vi "SpreadsheetFGV.vi"(6 "Message Ref":refnum<vi>, 7 "FGV Control":T1=enum."Init", 8 "Error In":errorcluster, 10 "Check -in Time":timestamp, 11 "Student ID":i32) -> (0 "Error Out":errorcluster, 1 "Checked In?":bool, 2 "Names":string[](array[string]), 3 "Message":string, 4 "Elapsed Time":i32)   [LabVIEW 2017]
uses:
  Controls/CSVFGVStates.ctl
  <vilib>/Utility/file.llb/Write To Spreadsheet File (string).vi
  <vilib>/Utility/file.llb/Read From Spreadsheet File (string).vi
panel:
  out "Output 2D Data":string[][](array[string])
  in  "CheckedInOutColumn":i32=3
  out "Checked In":string
  out "all rows":string[][](array[string])
  in  "Replacement":string
  in  "Student Names":i32(listbox)
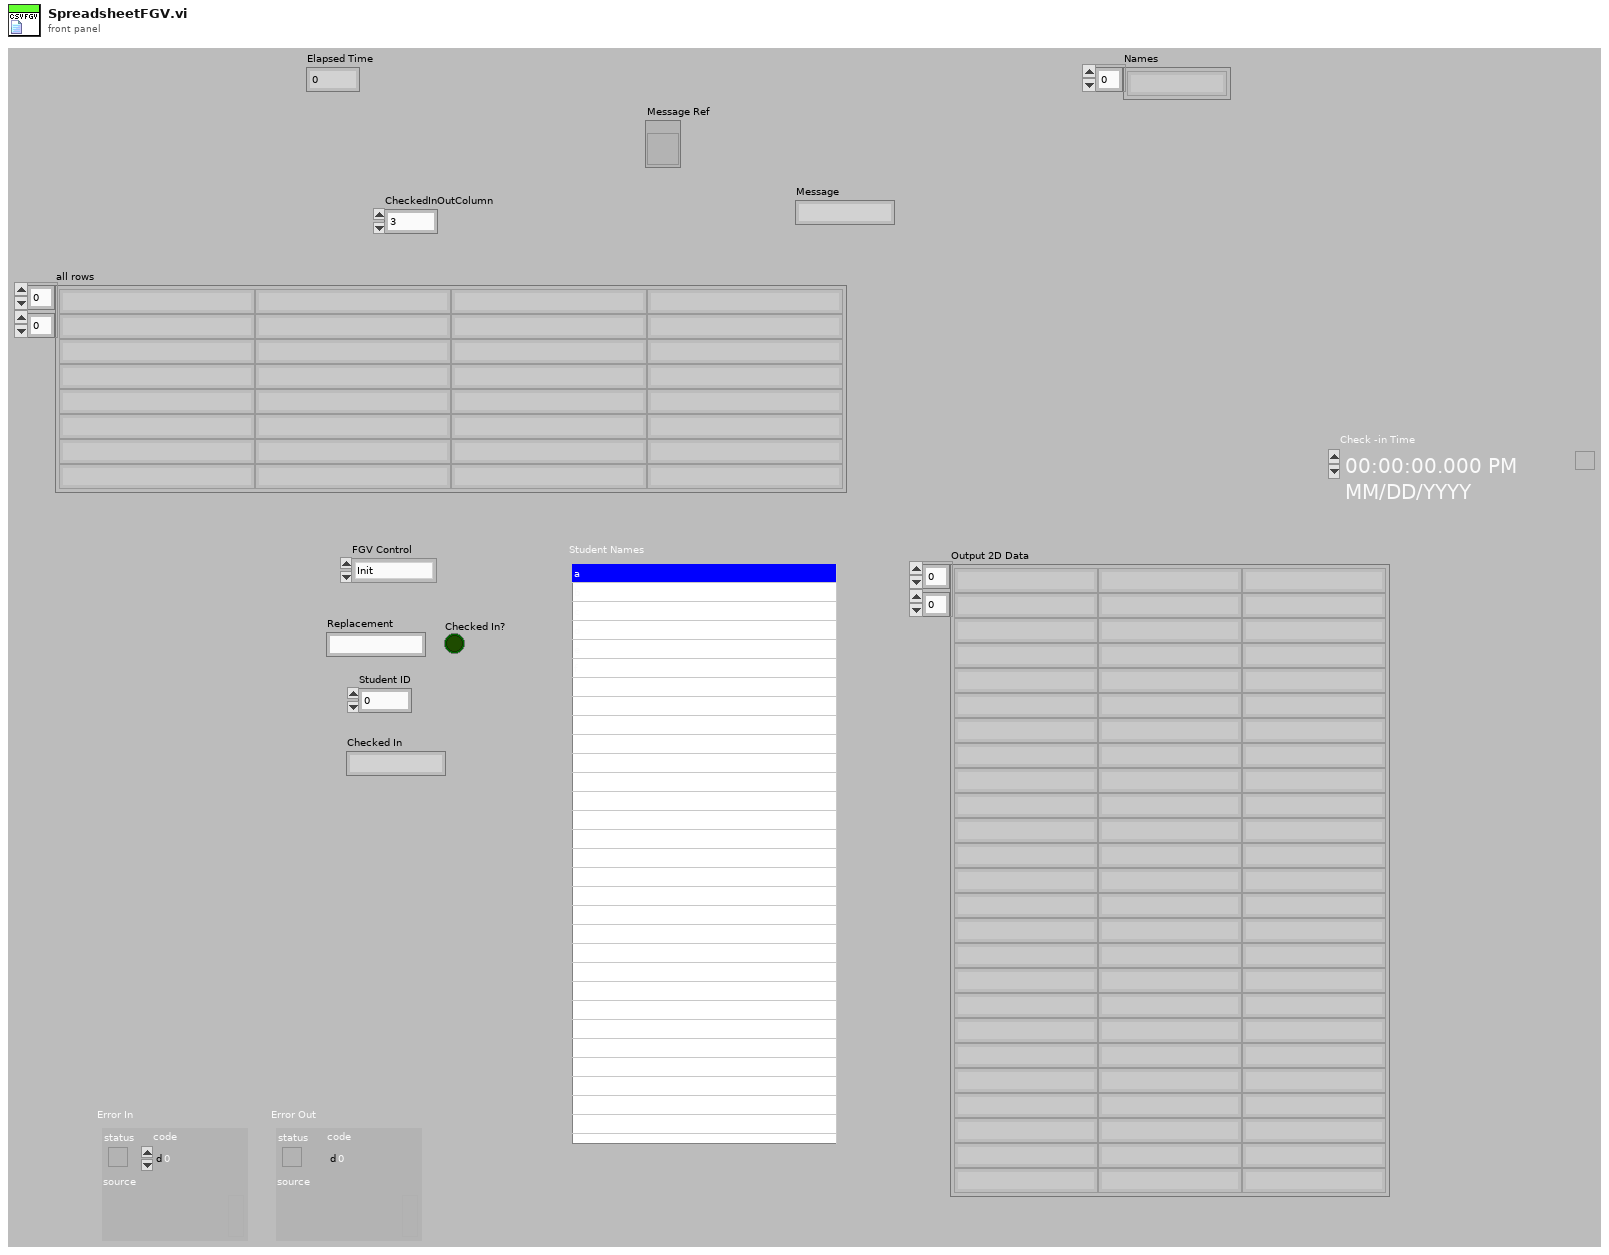
[diagram p1: front panel]
types:
  T1 = typedef "CSVFGVStates.ctl" = enum16{"Quit", "Init", "Sort", "Disable Camera", "Check In", "Check Out", "Check Status", "Read CSV", "Close Out"}
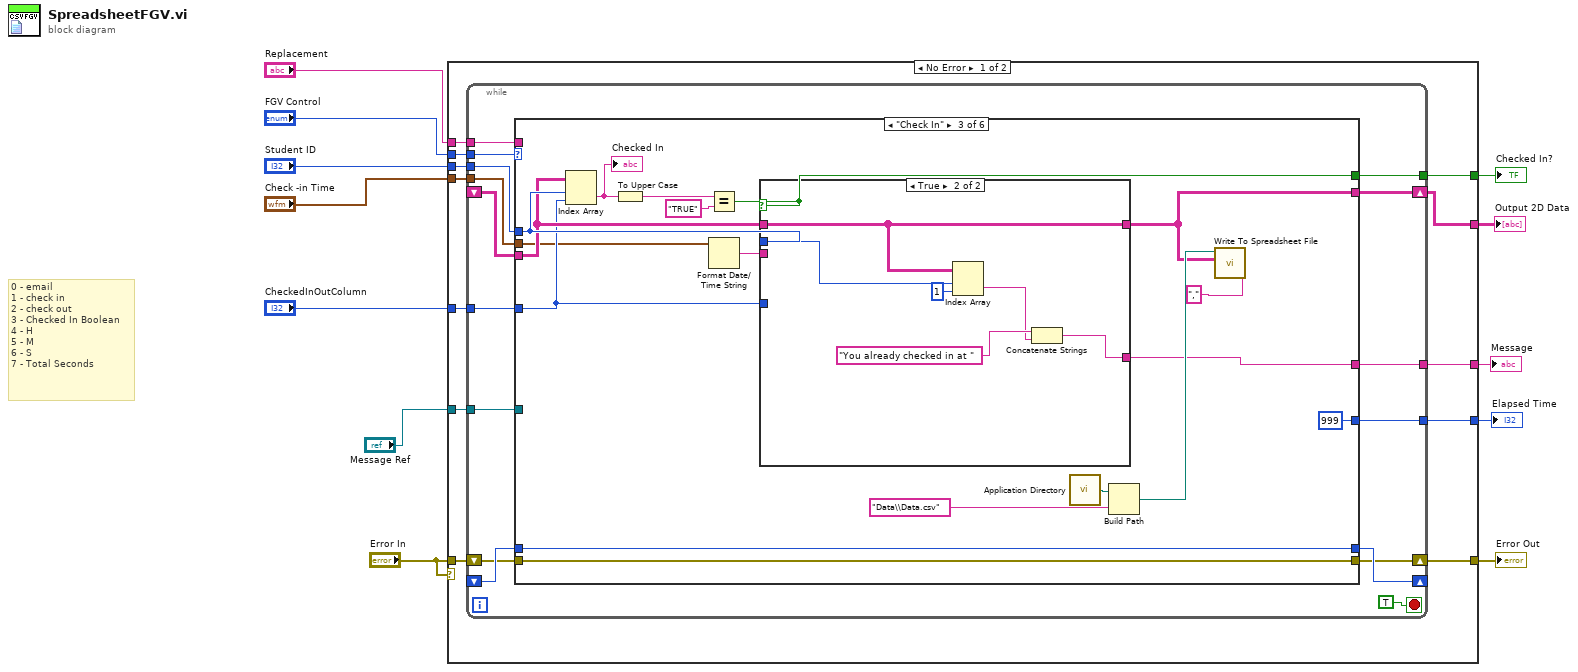
[diagram p0: block diagram]
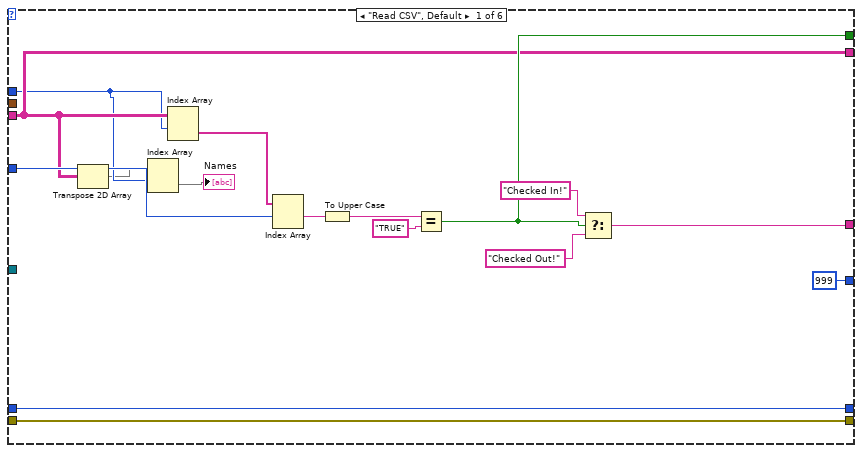
[diagram p2: hidden frame]
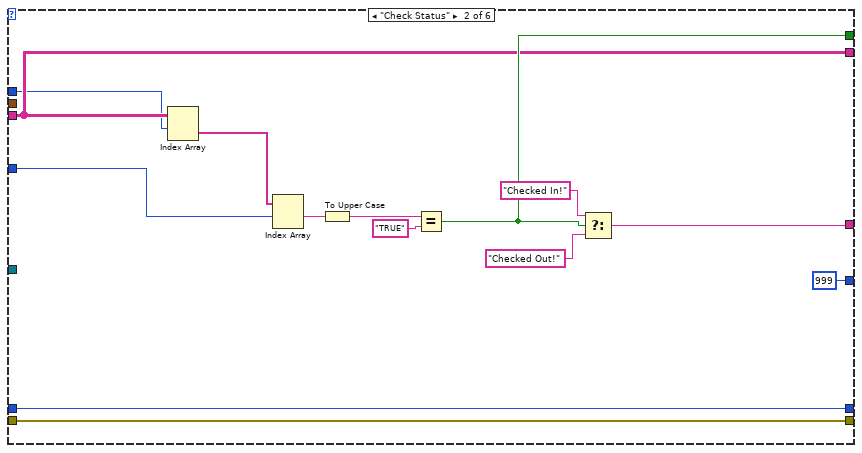
[diagram p3: hidden frame]
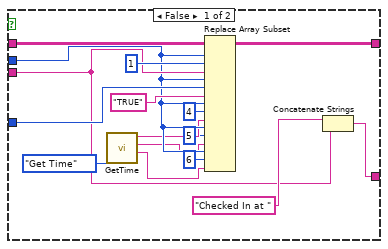
[diagram p4: hidden frame]
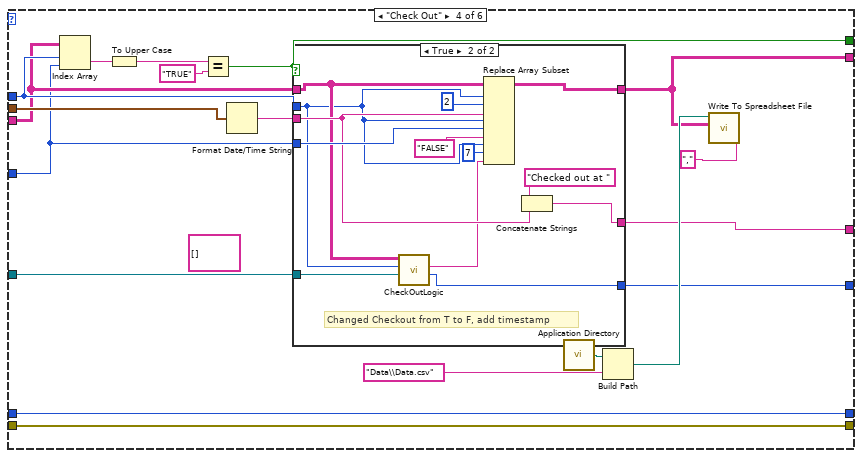
[diagram p5: hidden frame]
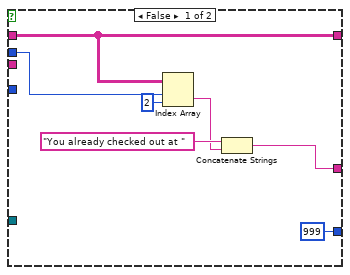
[diagram p6: hidden frame]
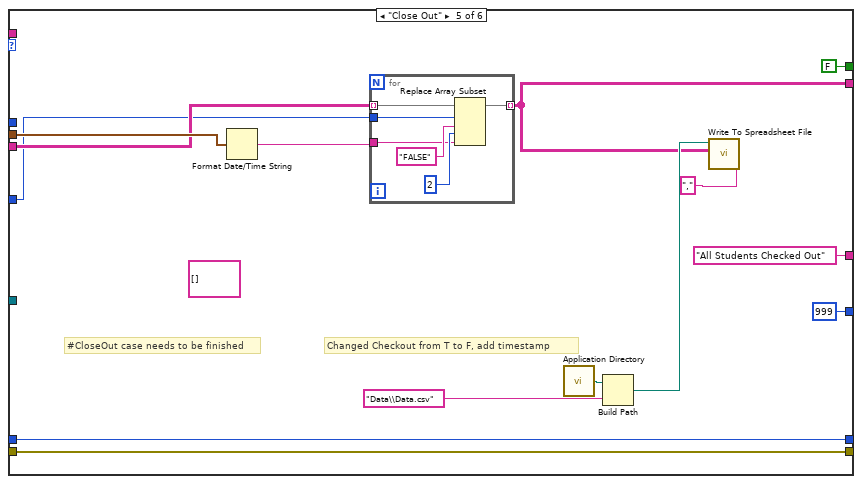
[diagram p7: hidden frame]
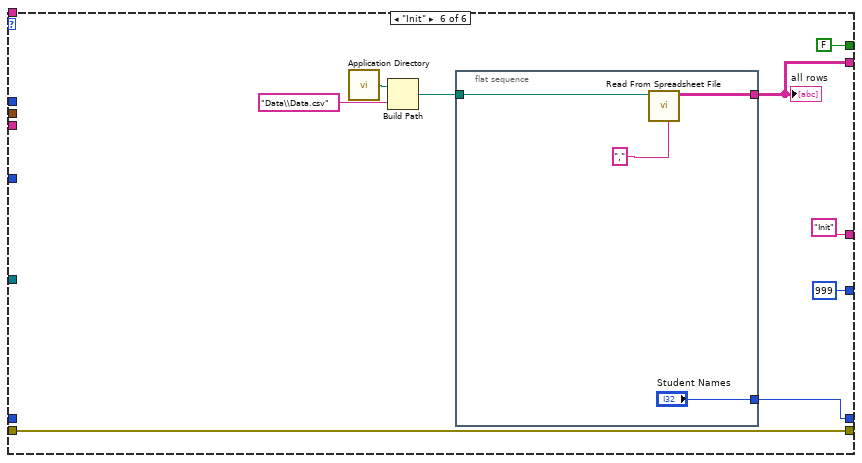
[diagram p8: hidden frame]
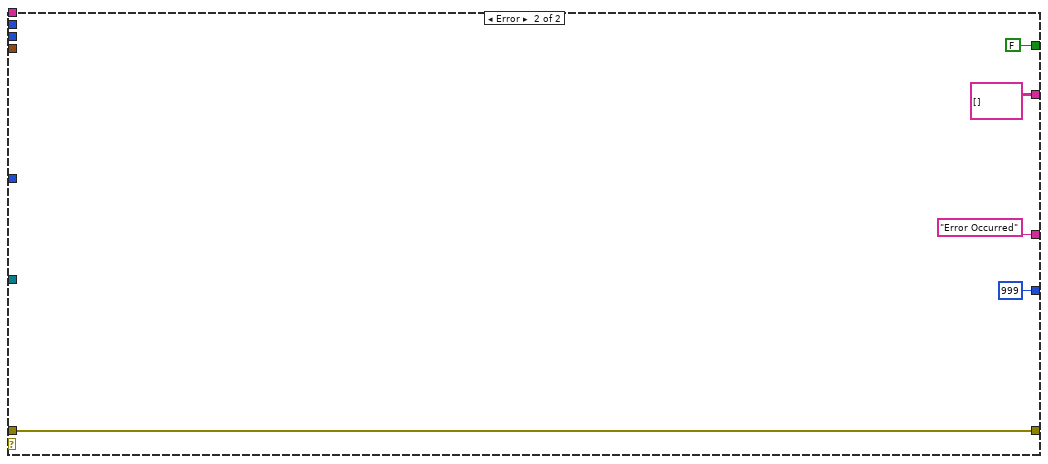
[diagram p9: hidden frame]
diagram:
  # "0 - email\n1 - check in\n2 - check out\n3 - Checked In Boolean\n4 - H\n5 - M\n6 - S\n7 - Total Seconds"
  n1 = case shown="No Error" "Error In" {
    tunnel: "FGV Control" -> [w24 _]
    tunnel: "Error In" -> [w22 w187]
    tunnel: [w23 w187] -> w10
    tunnel: "Student ID" -> [w21 _]
    tunnel: "Check -in Time" -> [w20 _]
    tunnel: "Replacement" -> [w19 _]
    tunnel: [w18 FALSE] -> w6
    tunnel: "CheckedInOutColumn" -> [w17 _]
    tunnel: [w16 string[][] [] ("all rows")] -> w4
    tunnel: [w15 "Error Occurred" ("date/time string")] -> w3
    tunnel: [w14 999 ("Elapsed Seconds")] -> w2
    tunnel: "Message Ref" -> [w13 _]
    frame No Error {
      n2 = while {
        shift-right: [w30] -> w16
        shift-left: _ -> [w38]
        tunnel: w24 -> [w39]
        shift-right: [w37] -> _
        shift-left: _ -> [w36]
        shift-right: [w35] -> w23
        shift-left: w22 -> [w34]
        tunnel: w21 -> [w33]
        tunnel: w20 -> [w32]
        tunnel: w19 -> [w31]
        tunnel: [w29] -> w18
        tunnel: w17 -> [w28]
        tunnel: [w27] -> w15
        tunnel: [w26] -> w14
        tunnel: w13 -> [w25]
        stop <- TRUE stop-if-true
        n3 = case shown="\"Check In\"" w39 {
          tunnel: w38 -> [w44 w58 w76 w116 w155 _]
          tunnel: [w55 w69 w84 w125 w159 w176] -> w37
          tunnel: w36 -> [w55 w69 w84 w125 w159 _]
          tunnel: [w56 w70 w86 w127 w161 w175] -> w35
          tunnel: w34 -> [w56 w70 w86 w127 w161 w175]
          tunnel: w33 -> [w43 w57 w77 w117 _ _]
          tunnel: w32 -> [_ _ w72 w123 w157 _]
          tunnel: w31 -> [_ _ _ _ _ _]
          tunnel: [w44 w58 w81 w121 w156 w174] -> w30
          tunnel: [w48 w62 w75 w115 FALSE FALSE] -> w29
          tunnel: w28 -> [w49 w63 w73 w114 w154 _]
          tunnel: [w45 w59 w74 w113 "All Students Checked Out" ("date/time string") "Init" ("date/time string")] -> w27
          tunnel: [999 ("Elapsed Seconds") 999 ("Elapsed Seconds") 999 ("Elapsed Seconds") w112 999 ("Elapsed Seconds") 999 ("Elapsed Seconds")] -> w26
          tunnel: w25 -> [_ _ _ w111 _ _]
          frame "Read CSV", Default {
            n4 = Transpose 2D Array(2D array=w44) -> (transposed array=w42:string[][])
            n5 = Index Array(array=w42, index (row)=w43) -> (element=→"Names":string[])  [unwired: 1 in]
            n6 = Index Array(array=w44, index (row)=w43) -> (element=w50:string[])  [unwired: 1 in]
            n7 = Index Array(array=w50, index #1=w49) -> (element #1=w53:string)  [unwired: 1 in, 1 out]
            n8 = To Upper Case(1:w53) -> (0:w52:string)
            n9 = Equal?(x=w52, y="TRUE") -> (x = y?=w48:bool)
            n10 = Select(t="Checked In!" ("y"), s=w48, f="Checked Out!" ("y")) -> (s? t:f=w45:string)
          }
          frame "Check Status" {
            n11 = Index Array(array=w58, index (row)=w57) -> (element=w64:string[])  [unwired: 1 in]
            n12 = Index Array(array=w64, index #1=w63) -> (element #1=w67:string)  [unwired: 1 in, 1 out]
            n13 = To Upper Case(1:w67) -> (0:w66:string)
            n14 = Equal?(x=w66, y="TRUE") -> (x = y?=w62:bool)
            n15 = Select(t="Checked In!" ("y"), s=w62, f="Checked Out!" ("y")) -> (s? t:f=w59:string)
          }
          frame "Check In" {
            n16 = Index Array(array=w76, index (row)=w77, index (col)=w73) -> (element=w80:string)
            "Checked In" <- w80
            n17 = To Upper Case(1:w80) -> (0:w79:string)
            n18 = Equal?(x=w79, y="TRUE") -> (x = y?=w75:bool)
            n19 = Format Date/Time String(seconds (now)=w72) -> (date/time string=w82:string)  [unwired: 2 in]
            n20 = case shown="True" w75 {
              tunnel: w82 -> [w98 _]
              tunnel: [w103 w110] -> w81
              tunnel: w77 -> [w96 w109]
              tunnel: w76 -> [w101 w110]
              tunnel: [w97 w105] -> w74
              tunnel: w73 -> [w100 _]
              frame False {
                n21 = call "GetTime.vi"("State"=enum16{"Get Time", "Calculate Differential"}."Get Time") -> ("Seconds"=w90:string, "Minutes"=w92:string, "Hours"=w94:string)  [unwired: 5 in, 3 out]
                n22 = Replace Array Subset(array=w101, new element #1=w98, index (row) #1=w96, index (col) #1=1 ("disabled index (col)"), new element #2="TRUE" ("new element/subarray"), index (row) #2=w96, index (col) #2=w100, new element #3=w94, index (row) #3=w96, index (col) #3=4 ("disabled index (col)"), new element #4=w92, index (row) #4=w96, index (col) #4=5 ("disabled index (col)"), new element #5=w90, index (row) #5=w96, index (col) #5=6 ("disabled index (col)")) -> (w103:string[][])
                n23 = Concatenate Strings("Checked In at " ("String"), w98) -> (w97:string)
              }
              frame True {
                n24 = Index Array(array=w110, index (row)=w109, index (col)=1 ("disabled index (col)")) -> (element=w106:string)
                n25 = Concatenate Strings("You already checked in at " ("delimiter (\\t)"), w106) -> (w105:string)
              }
            }
            n26 = call <vilib>:"Application Directory.vi"() -> ("Application Directory"=w88:path)
            n27 = Build Path(base path=w88, name or relative path="Data\\Data.csv") -> (appended path=w85:path)
            n28 = call-poly <vilib>:"Write To Spreadsheet File.vi"("delimiter (\\t)"="," ("delimiter (\\t)"), "2D data"=w81, "file path (dialog if empty)"=w85) -> ()  [unwired: 5 in, 1 out]
          }
          frame "Check Out" {
            (unwired) string[][] [] ("all rows")
            n29 = Index Array(array=w116, index (row)=w117, index (col)=w114) -> (element=w120:string)
            n30 = To Upper Case(1:w120) -> (0:w119:string)
            n31 = Equal?(x=w119, y="TRUE") -> (x = y?=w115:bool)
            n32 = Format Date/Time String(seconds (now)=w123) -> (date/time string=w122:string)  [unwired: 2 in]
            n33 = case shown="True" w115 {
              tunnel: w122 -> [_ w145]
              tunnel: [w136 w148] -> w121
              tunnel: w117 -> [w135 w141]
              tunnel: w116 -> [w136 w142]
              tunnel: [w131 w144] -> w113
              tunnel: w114 -> [_ w146]
              tunnel: [999 ("Elapsed Seconds") w138] -> w112
              tunnel: w111 -> [_ w137]
              frame False {
                n34 = Index Array(array=w136, index (row)=w135, index (col)=2 ("disabled index (col)")) -> (element=w132:string)
                n35 = Concatenate Strings("You already checked out at " ("string"), w132) -> (w131:string)
              }
              frame True {
                # "Changed Checkout from T to F, add timestamp"
                n36 = call "CheckOutLogic.vi"("Message Ref"=w137, "Student ID"=w141, "Student List In"=w142) -> ("Total Elapsed Time"=w138:i32, "Total Seconds Out"=w139:string)  [unwired: 2 in, 4 out]
                n37 = Replace Array Subset(array=w142, new element #1=w145, index (row) #1=w141, index (col) #1=2 ("disabled index (col)"), new element #2="FALSE" ("new element/subarray"), index (row) #2=w141, index (col) #2=w146, new element #3=w139, index (row) #3=w141, index (col) #3=7 ("disabled index (col)")) -> (w148:string[][])
                n38 = Concatenate Strings("Checked out at " ("string"), w145) -> (w144:string)
              }
            }
            n39 = call <vilib>:"Application Directory.vi"() -> ("Application Directory"=w129:path)
            n40 = Build Path(base path=w129, name or relative path="Data\\Data.csv") -> (appended path=w126:path)
            n41 = call-poly <vilib>:"Write To Spreadsheet File.vi"("delimiter (\\t)"="," ("delimiter (\\t)"), "2D data"=w121, "file path (dialog if empty)"=w126) -> ()  [unwired: 5 in, 1 out]
          }
          frame "Close Out" {
            (unwired) string[][] [] ("all rows")
            # "#CloseOut case needs to be finished"
            # "Changed Checkout from T to F, add timestamp"
            n42 = Format Date/Time String(seconds (now)=w157) -> (date/time string=w151:string)  [unwired: 2 in]
            n43 = for {
              tunnel: [w169] -> w156 mode=indexing
              tunnel: w155 -> [w168] mode=indexing
              tunnel: w154 -> [w167]
              tunnel: w151 -> [w164]
              n44 = Replace Array Subset(array=w168, new element #1="FALSE" ("new element/subarray"), index #1=w167, new element #2=w164, index #2=2 ("index")) -> (w169:string[])
            }
            n45 = call <vilib>:"Application Directory.vi"() -> ("Application Directory"=w163:path)
            n46 = Build Path(base path=w163, name or relative path="Data\\Data.csv") -> (appended path=w160:path)
            n47 = call-poly <vilib>:"Write To Spreadsheet File.vi"("delimiter (\\t)"="," ("delimiter (\\t)"), "2D data"=w156, "file path (dialog if empty)"=w160) -> ()  [unwired: 5 in, 1 out]
          }
          frame "Init" {
            n48 = call <vilib>:"Application Directory.vi"() -> ("Application Directory"=w178:path)
            n49 = Build Path(base path=w178, name or relative path="Data\\Data.csv") -> (appended path=w173:path)
            n50 = flat-sequence {
              tunnel: w173 -> [w182]
              tunnel: [w181] -> w174
              tunnel: ["Student Names"] -> w176
              frame #0 {
                n51 = call-poly <vilib>:"Read From Spreadsheet File.vi"("delimiter (\\t)"="," ("delimiter (\\t)"), "file path (dialog if empty)"=w182) -> ("all rows"=w181:string[][])  [unwired: 5 in, 4 out]
              }
            }
            "all rows" <- w174
          }
        }
      }
    }
    frame Error {
    }
  }
  "Error Out" <- w10
  "Checked In?" <- w6
  "Output 2D Data" <- w4
  "Message" <- w3
  "Elapsed Time" <- w2
